vi "Load Configuration.vi"(0 "INI Station Configuration in":refnum<class "Synchronize AWS S3 Content Station Configuration.lvclass">, 5 "INI file path in":path, 11 "error in":errorcluster) -> (4 "INI Station Configuration out":refnum<class "Synchronize AWS S3 Content Station Configuration.lvclass">, 15 "error out":errorcluster)   [LabVIEW 2026, in "Synchronize AWS S3 Content.lvlib" / "Synchronize AWS S3 Content Station Configuration.lvclass"]
uses:
  Synchronize AWS S3 Content Station Configuration.lvclass
  Synchronize AWS S3 Content Station Configuration.lvclass/Synchronize AWS S3 Content Station Configuration.ctl
  <vilib>/Utility/config.llb/Read Key (String).vi
  <vilib>/Utility/config.llb/NI_LVConfig.lvlib
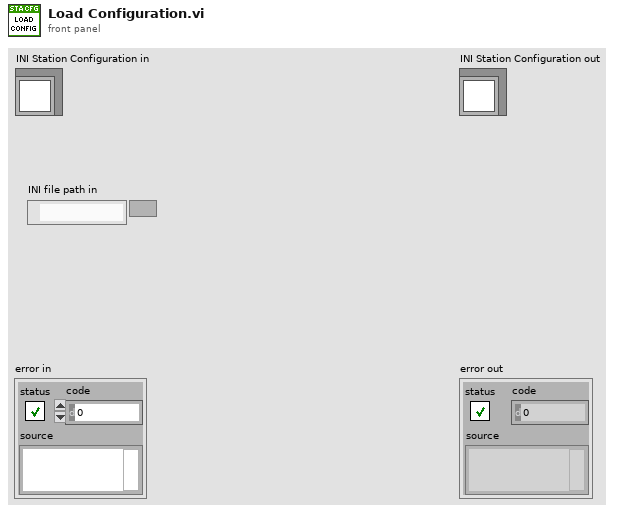
[diagram p1: front panel]
types:
  T1 = typedef "NI_LVConfig.lvlib/Config Data RefNum.ctl" = refnum<k1>
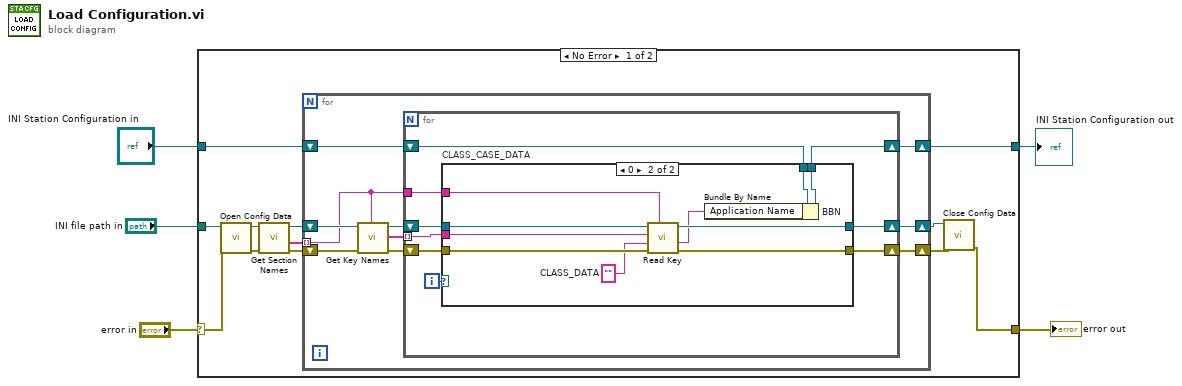
[diagram p0: block diagram]
diagram:
  n1 = case shown="No Error" "error in" {
    selector: "error in" -> [w14 w51]
    tunnel: [w17 w50] -> w2
    tunnel: [w10 w51] -> w1
    tunnel: "INI Station Configuration in" -> [w16 w50]
    tunnel: "INI file path in" -> [w15 _]
    frame No Error {
      n2 = call <vilib>:"Open Config Data.vi"("error in (no error)"=w14, "configuration file path"=w15) -> ("error out"=w6:errorcluster, "refnum"=w13:T1)  [unwired: 7 in, 1 out]
      n3 = call <vilib>:"Get Section Names.vi"("error in (no error)"=w6, "refnum"=w13) -> ("error out"=w7:errorcluster, "section names"=w8:string[], "refnum out"=w9:T1)  [unwired: 7 in]
      n4 = for {
        shift-right: [w27] -> w17
        shift-left: w16 -> [w26]
        shift-right: [w23] -> w11
        shift-left: w7 -> [w19]
        shift-right: [w24] -> w12
        shift-left: w9 -> [w25]
        tunnel: w8 -> [w21] mode=indexing
        n5 = call <vilib>:"Get Key Names.vi"("section"=w21, "error in (no error)"=w19, "refnum"=w25) -> ("error out"=w18:errorcluster, "key names"=w20:string[], "refnum out"=w22:T1)  [unwired: 5 in, 1 out]
        n6 = for {
          shift-right: [w35] -> w27
          shift-left: w26 -> [w30]
          shift-right: [w32] -> w23
          shift-left: w18 -> [w34]
          shift-right: [w31] -> w24
          shift-left: w22 -> [w33]
          tunnel: w21 -> [w29]
          tunnel: w20 -> [w28] mode=indexing
          i -> [w36]
          n7 = case "CLASS_CASE_DATA" shown="0" w36 {
            tunnel: [w37 w43] -> w35
            tunnel: w34 -> [w38 w48]
            tunnel: w33 -> [w39 w49]
            tunnel: [w38 w46] -> w32
            tunnel: [w39 w45] -> w31
            tunnel: w30 -> [w37 w40]
            tunnel: w29 -> [_ w42]
            tunnel: w28 -> [_ w41]
            frame Default {
            }
            frame 0 {
              w47 = ""  # CLASS_DATA
              n8 = call-poly <vilib>:"Read Key.vi"("section"=w42, "error in (no error)"=w48, "default value"=w47, "key"=w41, "refnum"=w49) -> ("error out"=w46:errorcluster, "value"=w44:string, "refnum out"=w45:T1)  [unwired: 3 in, 1 out]
              n9 = Bundle By Name "BBN"(cluster=w40, "Application Name"=w44) -> (w43:refnum<class "Synchronize AWS S3 Content Station Configuration.lvclass">)
            }
          }
        }
      }
      n10 = call <vilib>:"Close Config Data.vi"("error in (no error)"=w11, "refnum"=w12) -> ("error out"=w10:errorcluster)  [unwired: 8 in, 1 out]
    }
    frame Error {
    }
  }
  "error out" <- w1
  "INI Station Configuration out" <- w2
